vi "Request Data JSON.vi"(8 "error in (no error)":errorcluster, 11 "GetPersistentData in":refnum<class "GetPersistentData.lvclass">) -> (0 "error out":errorcluster, 2 "Request Data JSON":string, 3 "GetPersistentData out":refnum<class "GetPersistentData.lvclass">)   [LabVIEW 2020, in "obs-websocket.lvlib" / "GetPersistentData.lvclass"]
uses:
  GetPersistentData.lvclass
  GetPersistentData.lvclass/GetPersistentData.ctl
  <vilib>/IlluminatedG/lv-web-crypto/lv-json/JSON/JSON.lvlib
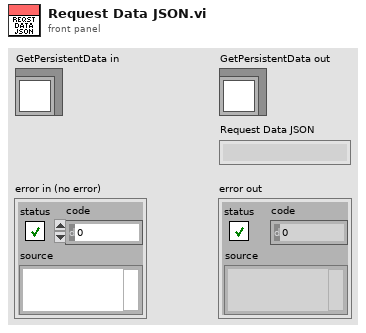
[diagram p1: front panel]
types:
  T1 = typedef "obs-websocket.lvlib/Data Realm.ctl" = enum16{"Global", "Profile"}
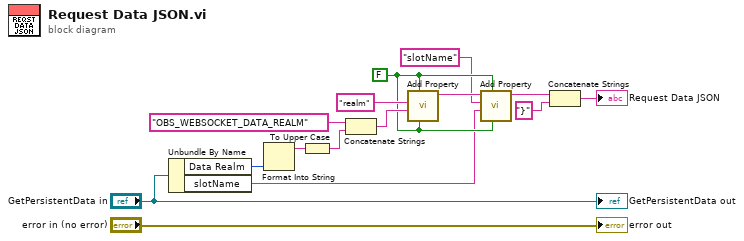
[diagram p0: block diagram]
diagram:
  w6 = FALSE ("Include Empty?")
  n1 = Unbundle By Name("GetPersistentData in") -> ("Data Realm"=w13:T1, "slotName"=w4:string)
  n2 = Format Into String(w13) -> (resulting string=w12:string)  [unwired: 3 in, 1 out]
  n3 = To Upper Case(1:w12) -> (0:w11:string)
  n4 = Concatenate Strings("OBS_WEBSOCKET_DATA_REALM" ("string"), w11) -> (w8:string)
  n5 = call <vilib>:"Add Property.vi"("String?"=w6, "Include Empty?"=w6, "Value"=w8, "Property Name"="realm") -> ("String out"=w7:string)  [unwired: 7 in]
  n6 = call <vilib>:"Add Property.vi"("String?"=w6, "Include Empty?"=w6, "Value"=w4, "Property Name"="slotName", "String In"=w7) -> ("String out"=w3:string)  [unwired: 6 in]
  n7 = Concatenate Strings(w3, "}" ("string")) -> (→"Request Data JSON":string)
  "error out" <- "error in (no error)"
  "GetPersistentData out" <- "GetPersistentData in"
